vi "Lift Joystick Get Arrays.vi"(8 "Button Index's":T2, 9 "Setpoints":T1, 10 "Joystick IN":bool[](array[boolean]), 11 "Position IN":dbl format="%#_13g") -> (2 "Which Button?":i32, 3 "Position":dbl)   [LabVIEW 2014]
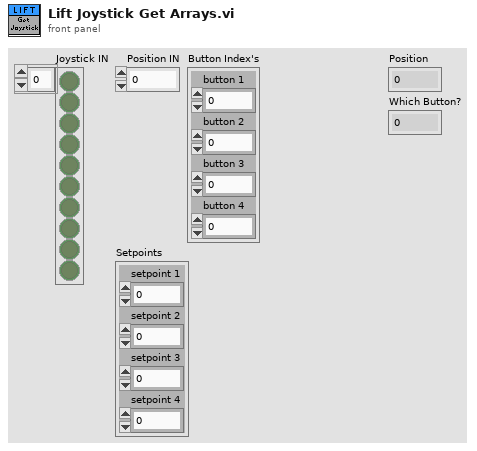
[diagram p1: front panel]
types:
  T1 = cluster{"setpoint 1":dbl, "setpoint 2":dbl, "setpoint 3":dbl, "setpoint 4":dbl}
  T2 = cluster{"button 1":i32, "button 2":i32, "button 3":i32, "button 4":i32}
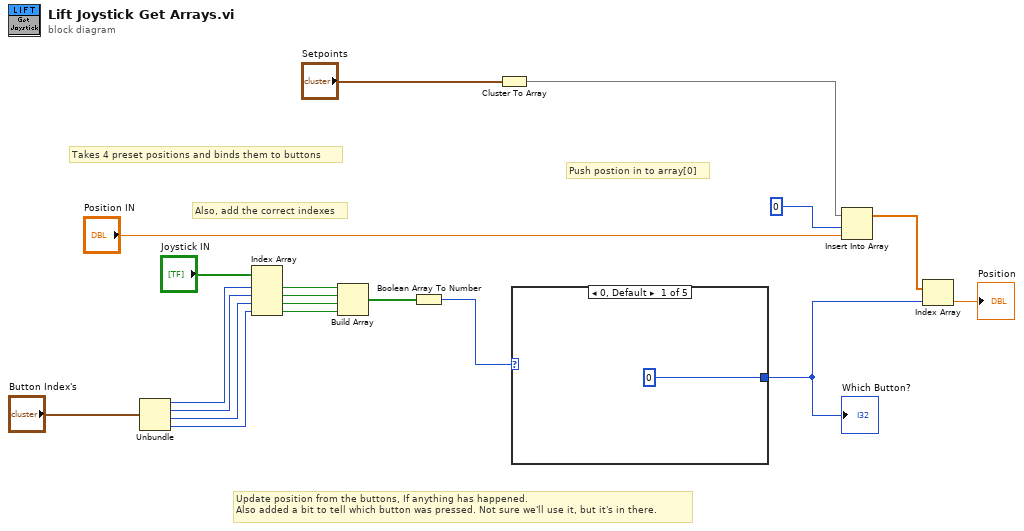
[diagram p0: block diagram]
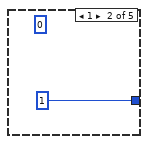
[diagram p2: hidden frame]
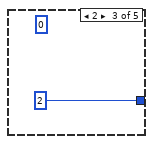
[diagram p3: hidden frame]
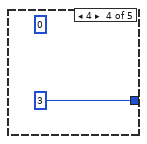
[diagram p4: hidden frame]
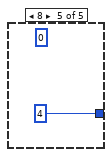
[diagram p5: hidden frame]
diagram:
  # "Push postion in to array[0]"
  # "Takes 4 preset positions and binds them to buttons"
  # "Update position from the buttons, If anything has happened.\nAlso added a bit to tell which button was pressed. Not sure we'll use it, but it's in there."
  # "Also, add the correct indexes"
  n1 = Unbundle("Button Index's") -> ("button 1"=w17:i32, "button 2"=w16:i32, "button 3"=w15:i32, "button 4"=w14:i32)
  n2 = Index Array(array="Joystick IN", index #1=w17, index #2=w16, index #3=w15, index #4=w14) -> (element #1=w10:bool, element #2=w11:bool, element #3=w12:bool, element #4=w13:bool)
  n3 = Build Array(w10, w11, w12, w13) -> (w9:bool[])
  n4 = Boolean Array To Number(Boolean array=w9) -> (number=w8:u32)
  n5 = Cluster To Array(cluster="Setpoints") -> (array=w6:dbl[])
  n6 = case shown="0, Default" w8 {
    tunnel: [0 1 2 3 4] -> w3
    frame 0, Default {
    }
    frame 1 {
      (unwired) 0
    }
    frame 2 {
      (unwired) 0
    }
    frame 4 {
      (unwired) 0
    }
    frame 8 {
      (unwired) 0
    }
  }
  "Which Button?" <- w3
  n7 = Insert Into Array(array=w6, index=0, new element="Position IN") -> (w2:dbl[])
  n8 = Index Array(array=w2, index=w3) -> (element=→"Position":dbl)
